vi "SetParameters.vi"(8 "error in (no error)":errorcluster, 9 "Parameters":string, 11 "CGrapherDGML in":refnum<class "CGrapherDGML.lvclass">) -> (0 "error out":errorcluster, 3 "CGrapherDGML out":refnum<class "CGrapherDGML.lvclass">)   [LabVIEW 2020, in "DefaultExtensions.lvlib" / "CGrapherDGML.lvclass"]
uses:
  CGrapherDGML.lvclass
  Private/Parameters.ctl
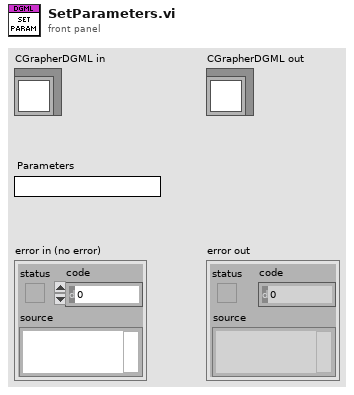
[diagram p1: front panel]
types:
  T1 = typedef "DefaultExtensions.lvlib/CGrapherDGML.lvclass/Parameters.ctl" = cluster{"Path":string, "Expand containers":bool, "Group by folder":bool, "Show full paths":bool, "Source folder?":bool, "Target folder?":bool}
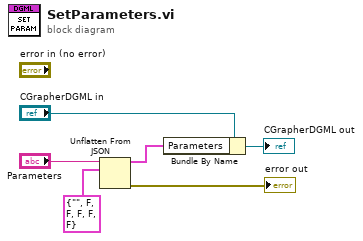
[diagram p0: block diagram]
diagram:
  n1 = Unflatten From JSON(JSON string="Parameters", type and defaults=T1 {"Path"="", "Expand containers"=FALSE, "Group by folder"=FALSE, "Show full paths"=FALSE, "Source folder?"=FALSE, "Target folder?"=FALSE} ("Parameters")) -> (value=w2:T1, error out=→"error out":errorcluster)  [unwired: 5 in]
  n2 = Bundle By Name(cluster="CGrapherDGML in", "Parameters"=w2) -> (→"CGrapherDGML out":refnum<class "CGrapherDGML.lvclass">)
